vi "newmain.vi"() -> ()   [LabVIEW 2018]
uses:
  INPUTS.ctl
  <vilib>/DAQmx/read.llb/DAQmx Read (Analog 2D DBL NChan NSamp).vi
  <vilib>/DAQmx/configure/timing.llb/DAQmx Timing (Sample Clock).vi
  <vilib>/Utility/file.llb/Read Delimited Spreadsheet (DBL).vi
  <vilib>/DAQmx/miscellaneous.llb/DAQmx Fill In Error Info.vi
  <instrlib>/Kikusui PLZ 4W Series/Kikusui PLZ 4W Series.lvlib
  <instrlib>/Agilent E4360/Agilent E4360.lvlib
panel:
  out "Power":cluster{dbl[], dbl[]}[](graph) caption="VCC"
  out "P_CELL":dbl format="%0.3f"
  out "P_PV":dbl format="%0.3f"
  out "P_LOAD":dbl format="%0.3f"
  in  "DET or PPT?":enum16{"DET", "PPT"}(ring)
  out "Elapsed":dbl format="%#_13g"
  in  "SAS file":path=path "C:/Repository/bdc_prototype/logger/pcosplot.csv"
  in  "SAS VISA":refnum<visa-resource-name>="USB0::0x0957::0x1107::MY54001612::INSTR"
  in  "Load connected to?":enum16{"V_BUS", "V_CELL"}(ring)
  in  "ELO file":path=path "C:/Repository/bdc_prototype/logger/cp_profile.csv"
  in  "Serial Configuration":cluster{"Baud Rate":u32, "Stop Bits":u16}={"Baud Rate"=19200, "Stop Bits"=20} {"Stop Bits" items=["1.0"=10, "2.0"=20]; "Baud Rate" items=["2400"=2400, "4800"=4800, "9600"=9600, "19200"=19200]}
  in  "ELO VISA":refnum<visa-resource-name>="USB0::0x0B3E::0x1019::YL002399::INSTR"
  out "V_CC":dbl format="%0.3f"
  in  "Time (sec)":dbl=5560.0
  out "new file path (Not A Path if cancelled)":path
  out "I_CELL":dbl format="%0.3f"
  out "I_LOAD":dbl format="%0.3f"
  out "I_PV":dbl format="%0.3f"
  out "V_CELL":dbl format="%0.3f"
  out "V_BUS":dbl format="%0.3f"
  out "Currents":cluster{dbl[], dbl[]}[](graph) caption="VCC"
  out "Voltages":cluster{dbl[], dbl[]}[](graph) caption="VCC"
  in  "stop":bool
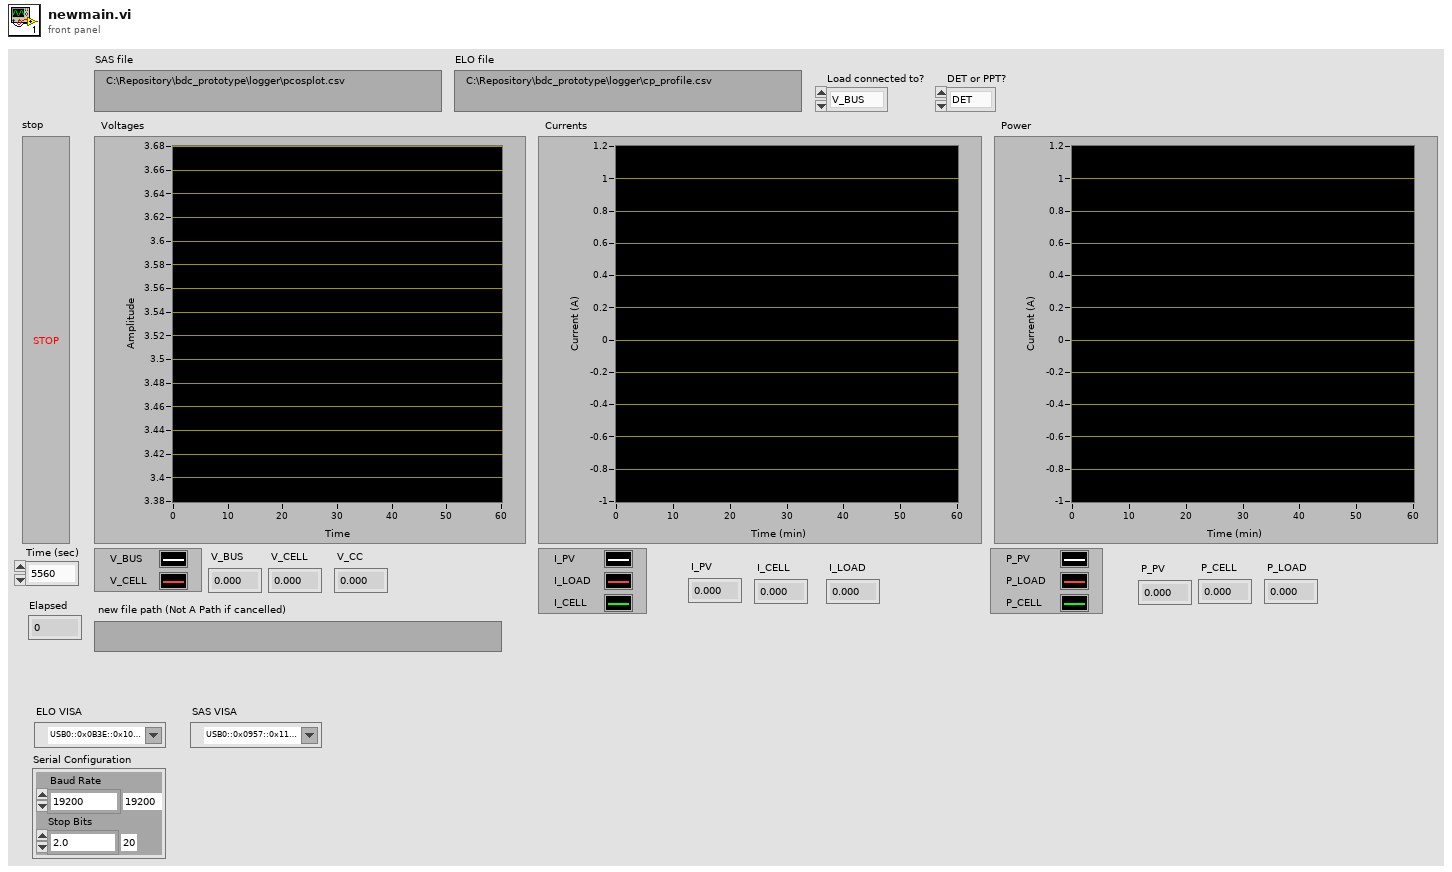
[diagram p1: front panel]
types:
  T1 = enum16{"open", "open or create", "create or replace", "create", "open (read only)"}
  T2 = typedef "INPUTS.ctl" = enum16{"VCC", "I_PV", "I_LOAD", "I_CELL", "V_BUS", "V_CELL", "I_LOAD2"}
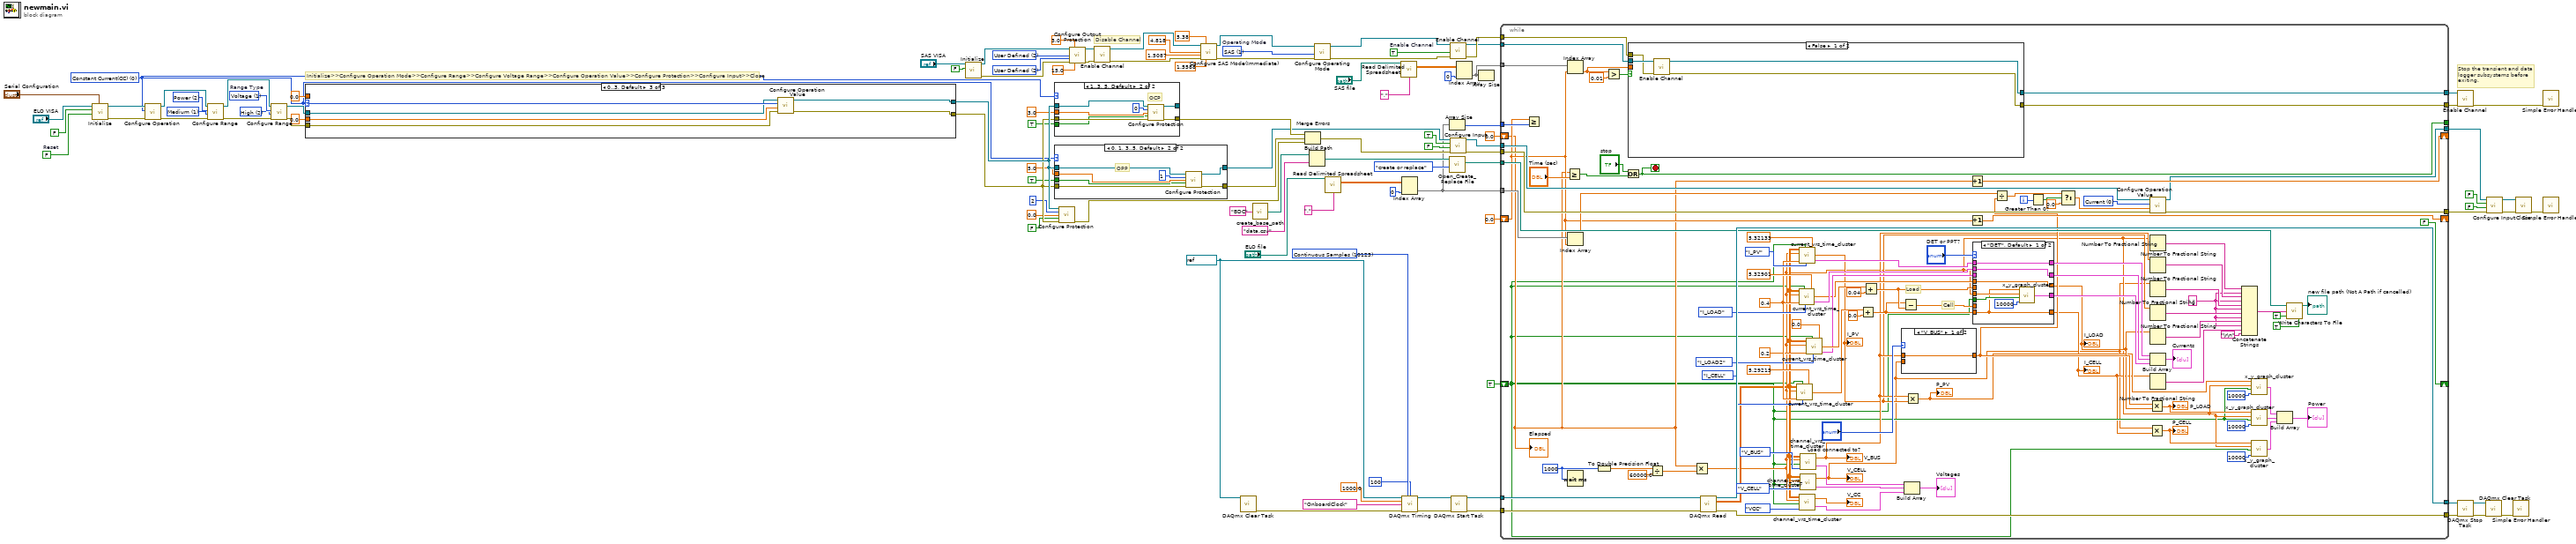
[diagram p0: block diagram]
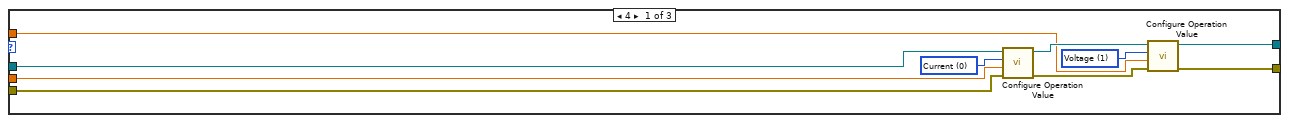
[diagram p4: hidden frame]
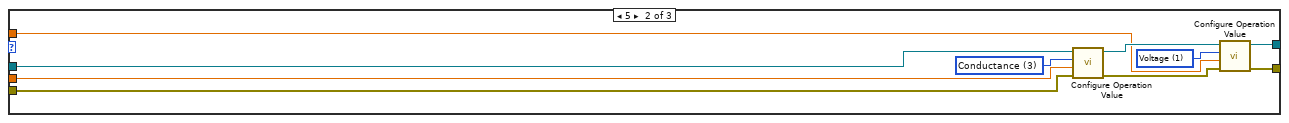
[diagram p5: hidden frame]
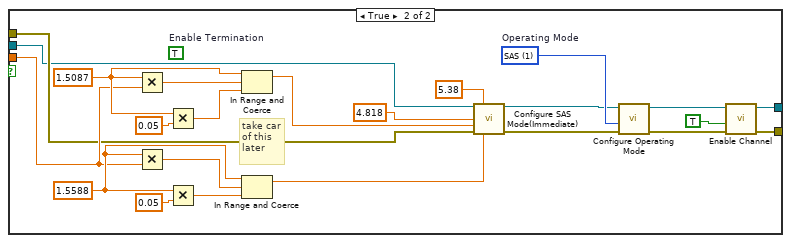
[diagram p6: hidden frame]
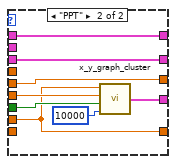
[diagram p7: hidden frame]
diagram:
  w25 = 2 items=["MAX", "MIN", "User Defined"] ("Voltage Limit Source (0:MAX)")
  w26 = 2 items=["MAX", "MIN", "User Defined"] ("Current Limit Source (0:MAX)")
  w31 = TRUE  # Enable Channel
  w32 = 1 items=["Fixed", "SAS", "Table"]  # Operating Mode
  w52 = u16 2 items=["Current", "Voltage", "Power", "Conductance"] ("Range Type (0:Current)")
  w72 = u16 2 items=["Low"=0, "High"=2] ("Voltage Range (0:Low)")
  w71 = u16 1 items=["Low", "Medium", "High"] ("Input Range (0:Low)")
  w44 = u16 0 items=["Constant Current(CC)", "Constant Voltage(CV)", "Constant Power(CP)", "Constant Resistance(CR)", "Constant Current & Voltage(CCCV)", "Constant Resistance & Voltage(CRCV)"] ("Operation Mode (0:Constant Current)")
  w56 = FALSE  # Reset
  w73 = u16 1 items=["Current", "Voltage", "Power", "Conductance"]  # Range Type
  w86 = refnum<k21> "MEAS" ("task in")
  w105 = 10123 items=["Finite Samples"=10178, "Continuous Samples"=10123, "Hardware Timed Single Point"=12522] ("sample mode")
  # "Stop the transient and data logger subsystems before exiting."
  # "Disable Channel"
  # "Initialize>>Configure Operation Mode>>Configure Range>>Configure Voltage Range>>Configure Operation Value>>Configure Protection>>Configure Input>>Close"
  n1 = call <instrlib>:"Initialize.vi"("Serial Configuration"="Serial Configuration", "Reset (True)"=w56, "ID Query (True)"=FALSE, "VISA resource name"="ELO VISA") -> ("error out"=w80:errorcluster, "VISA resource name out"=w81:refnum<visa-resource-name>)  [unwired: 6 in]
  n2 = call <instrlib>:"Configure Operation.vi"("error in (no error)"=w80, "Operation Mode (0:Constant Current)"=w44, "VISA resource name"=w81) -> ("error out"=w74:errorcluster, "VISA resource name out"=w75:refnum<visa-resource-name>)  [unwired: 7 in]
  n3 = call <instrlib>:"Configure Range.vi"("error in (no error)"=w74, "Range (0:Low)"=w71, "Range Type (0:Current)"=w52, "VISA resource name"=w75) -> ("error out"=w76:errorcluster, "VISA resource name out"=w77:refnum<visa-resource-name>)  [unwired: 6 in]
  n4 = call <instrlib>:"Configure Range.vi"("error in (no error)"=w76, "Range (0:Low)"=w72, "Range Type (0:Current)"=w73, "VISA resource name"=w77) -> ("error out"=w78:errorcluster, "VISA resource name out"=w79:refnum<visa-resource-name>)  [unwired: 6 in]
  n5 = case shown="0..3, Default" w44 {
    selector: w44 -> [_ _ w129]
    tunnel: 0.0 ("Input Value(0)") -> [w111 w119 w132]
    tunnel: w79 -> [w116 w124 w128]
    tunnel: w78 -> [w115 w123 w127]
    tunnel: [w112 w122 w131] -> w70
    tunnel: [w109 w121 w130] -> w69
    tunnel: 0.0 ("Voltage Value (0)") -> [w110 w120 _]
    frame 4 {
      w107 = u16 1 items=["Current", "Voltage", "Power", "Conductance"] ("Value Type (0:Current)")
      w108 = u16 0 items=["Current", "Voltage", "Power", "Conductance"] ("Value Type (0:Current)")
      n6 = call <instrlib>:"Configure Operation Value.vi"("error in (no error)"=w115, "Values (0)"=w111, "Value Type (0:Current)"=w108, "VISA resource name"=w116) -> ("error out"=w113:errorcluster, "VISA resource name out"=w114:refnum<visa-resource-name>)  [unwired: 6 in]
      n7 = call <instrlib>:"Configure Operation Value.vi"("error in (no error)"=w113, "Values (0)"=w110, "Value Type (0:Current)"=w107, "VISA resource name"=w114) -> ("error out"=w109:errorcluster, "VISA resource name out"=w112:refnum<visa-resource-name>)  [unwired: 6 in]
    }
    frame 5 {
      w117 = u16 1 items=["Current", "Voltage", "Power", "Conductance"] ("Value Type (0:Current)")
      w118 = u16 3 items=["Current", "Voltage", "Power", "Conductance"] ("Value Type (0:Current)")
      n8 = call <instrlib>:"Configure Operation Value.vi"("error in (no error)"=w123, "Values (0)"=w119, "Value Type (0:Current)"=w118, "VISA resource name"=w124) -> ("error out"=w125:errorcluster, "VISA resource name out"=w126:refnum<visa-resource-name>)  [unwired: 6 in]
      n9 = call <instrlib>:"Configure Operation Value.vi"("error in (no error)"=w125, "Values (0)"=w120, "Value Type (0:Current)"=w117, "VISA resource name"=w126) -> ("error out"=w121:errorcluster, "VISA resource name out"=w122:refnum<visa-resource-name>)  [unwired: 6 in]
    }
    frame 0..3, Default {
      n10 = call <instrlib>:"Configure Operation Value.vi"("error in (no error)"=w127, "Values (0)"=w132, "Value Type (0:Current)"=w129, "VISA resource name"=w128) -> ("error out"=w130:errorcluster, "VISA resource name out"=w131:refnum<visa-resource-name>)  [unwired: 6 in]
    }
  }
  n11 = call <instrlib>:"Initialize.vi"("ID Query (True)"=FALSE, "VISA resource name"="SAS VISA") -> ("error out"=w29:errorcluster, "VISA resource name out"=w30:refnum<visa-resource-name>)  [unwired: 8 in]
  n12 = case shown="1..3, 5, Default" w44 {
    tunnel: w70 -> [w134 w141]
    tunnel: w69 -> [w133 w140]
    tunnel: [w134 w139] -> _
    tunnel: [w133 w138] -> w68
    tunnel: 3.0 ("OCP Limit (0)") -> [_ w137]
    tunnel: TRUE ("OCP Trip (Disable)") -> [_ w135]
    frame 0, 4 {
    }
    frame 1..3, 5, Default {
      # "OCP"
      n13 = call <instrlib>:"Configure Protection.vi"("VISA resource name"=w141, "Protection Type (0:OCP)"=0, "Protection Limit (0)"=w137, "Enable Trip (Disable)"=w135, "error in (no error)"=w140) -> ("VISA resource name out"=w139:refnum<visa-resource-name>, "error out"=w138:errorcluster)  [unwired: 9 in]
    }
  }
  n14 = case shown="0, 1, 3..5, Default" w44 {
    tunnel: w70 -> [w143 w150]
    tunnel: w69 -> [w142 w149]
    tunnel: [w143 w148] -> w65
    tunnel: [w142 w147] -> w58
    tunnel: 5.0 ("OPP Limit (0)") -> [_ w146]
    tunnel: TRUE ("OPP Trip (Disable)") -> [_ w144]
    frame 2 {
    }
    frame 0, 1, 3..5, Default {
      # "OPP"
      n15 = call <instrlib>:"Configure Protection.vi"("VISA resource name"=w150, "Protection Type (0:OCP)"=1, "Protection Limit (0)"=w146, "Enable Trip (Disable)"=w144, "error in (no error)"=w149) -> ("VISA resource name out"=w148:refnum<visa-resource-name>, "error out"=w147:errorcluster)  [unwired: 9 in]
    }
  }
  n16 = call <instrlib>:"Configure Protection.vi"("VISA resource name"=w70, "Protection Type (0:OCP)"=2, "Protection Limit (0)"=0.0 ("UVP Limit (0)"), "Enable Trip (Disable)"=FALSE ("UVP (Enable)"), "error in (no error)"=w69) -> ("error out"=w67:errorcluster)  [unwired: 9 in, 1 out]
  n17 = call <instrlib>:"Configure Output Protection.vi"("VISA resource name"=w30, "Current Limit (0 A)"=3.0, "Current Limit Source (0:MAX)"=w26, "Voltage Limit Source (0:MAX)"=w25, "error in (no error)"=w29, "Voltage Limit (0 V)"=15.0) -> ("VISA resource name out"=w16:refnum<visa-resource-name>, "error out"=w15:errorcluster)  [unwired: 8 in]
  n18 = call <instrlib>:"Enable Channel.vi"("error in (no error)"=w15, "VISA resource name"=w16) -> ("error out"=w23:errorcluster, "VISA resource name out"=w24:refnum<visa-resource-name>)  [unwired: 8 in]
  n19 = call <instrlib>:"Configure SAS Mode(Immediate).vi"("VISA resource name"=w24, "Open Circuit Voltage (0.0 V)"=5.38, "Maximum Voltage Point (0.0 V)"=4.818, "Maximum Current Point (0.0 A)"=1.5087, "error in (no error)"=w23, "Short Circuit Current (0.0 A)"=1.5588) -> ("VISA resource name out"=w18:refnum<visa-resource-name>, "error out"=w17:errorcluster)  [unwired: 8 in]
  n20 = call <vilib>:"DAQmx Clear Task.vi"("task in"=w86) -> ("error out"=w85:errorcluster)  [unwired: 14 in]
  n21 = call "create_base_path.vi"("project name"="BDC") -> ("base path"=w89:path)
  n22 = Merge Errors(w68, w58, w67) -> (w66:errorcluster)
  n23 = Build Path(base path=w89, name or relative path="data.csv") -> (appended path=w91:path)
  n24 = call <instrlib>:"Configure Operating Mode.vi"("error in (no error)"=w17, "Operating Mode (0:Fixed)"=w32, "VISA resource name"=w18) -> ("error out"=w13:errorcluster, "VISA resource name out"=w14:refnum<visa-resource-name>)  [unwired: 7 in]
  n25 = call-poly <vilib>:"Read Delimited Spreadsheet.vi"("file path (dialog if empty)"="ELO file", "delimiter (\\t)"="," ("delimiter (\\t)")) -> ("all rows"=w47:dbl[][])  [unwired: 8 in, 5 out]
  n26 = call-poly <vilib>:"Read Delimited Spreadsheet.vi"("file path (dialog if empty)"="SAS file", "delimiter (\\t)"="," ("delimiter (\\t)")) -> ("all rows"=w8:dbl[][])  [unwired: 8 in, 5 out]
  n27 = Index Array(array=w47, index (col)=0 ("disabled index (col)")) -> (element=w43:dbl[])  [unwired: 1 in]
  n28 = call-poly <vilib>:"DAQmx Timing.vi"("task/channels in"=w86, "sample mode"=w105, "samples per channel"=100, "rate"=1000.0, "source"=tag "OnboardClock", "error in"=w85) -> ("task out"=w102:refnum<k21>, "error out"=w101:errorcluster)  [unwired: 8 in]
  n29 = Array Size(array=w43) -> (size(s)=w42:i32)
  n30 = call <vilib>:"Open_Create_Replace File.vi"("function (open:0)"=T1."create or replace", "file path"=w91) -> ("new file path"=w87:path)  [unwired: 6 in, 3 out]
  n31 = call <instrlib>:"Enable Channel.vi"("error in (no error)"=w13, "Enable Channel (Disable)"=w31, "VISA resource name"=w14) -> ("error out"=w6:errorcluster, "VISA resource name out"=w5:refnum<visa-resource-name>)  [unwired: 7 in]
  n32 = call <instrlib>:"Configure Input.vi"("error in (no error)"=w66, "Enable Input Short (Disable)"=FALSE, "Enable Input (Enable)"=TRUE, "VISA resource name"=w65) -> ("error out"=w45:errorcluster, "VISA resource name out"=w46:refnum<visa-resource-name>)  [unwired: 6 in]
  n33 = call <vilib>:"DAQmx Start Task.vi"("task/channels in"=w102, "error in"=w101) -> ("task out"=w100:refnum<k21>, "error out"=w99:errorcluster)  [unwired: 12 in]
  n34 = Index Array(array=w8, index (col)=0 ("disabled index (col)")) -> (element=w7:dbl[])  [unwired: 1 in]
  n35 = Array Size(array=w7) -> ()  [unwired: 1 out]
  n36 = while {
    shift-right: [w224] -> _
    shift-left: 0.0 -> [w172]
    shift-right: [FALSE ("Clear Graph?")] -> _
    shift-left: TRUE ("Clear Graph?") -> [w155]
    tunnel: w100 -> [w250]
    tunnel: w99 -> [w249]
    tunnel: [w248] -> w98
    tunnel: [w247] -> w97
    tunnel: w87 -> [w225]
    tunnel: [w218] -> _
    tunnel: w46 -> [w209]
    tunnel: w45 -> [w208]
    tunnel: w43 -> [w207]
    tunnel: w42 -> [w206]
    tunnel: [w205] -> w36
    tunnel: [w204] -> w35
    shift-right: [w196] -> _
    shift-left: 0.0 -> [w194]
    tunnel: w7 -> [w195]
    tunnel: w6 -> [w193]
    tunnel: w5 -> [w192]
    tunnel: [w191] -> w3
    tunnel: [w190] -> w2
    i -> [w198]
    stop <- w218 stop-if-true
    w210 = u16 0 items=["Current", "Voltage", "Power", "Conductance"] ("Value Type (0:Current)")
    w228 = "," ("string")
    w211 = 0.4 ("sensitivity (V/A)")
    w251 = u32 1000 ("milliseconds to wait")
    # "Cell"
    # "Load"
    n37 = Greater Or Equal?(x=w194, y=w206) -> ()  [unwired: 1 out]
    n38 = Greater Or Equal?(x=w172, y="Time (sec)") -> (x >= y?=w219:bool)
    n39 = Index Array(array=w195, index=w194) -> (element=w170:dbl)
    n40 = Index Array(array=w207, index=w194) -> (element=w203:dbl)
    n41 = Wait (ms)(milliseconds to wait=w251) -> ()  [unwired: 1 out]
    n42 = To Double Precision Float(number=w251) -> (double precision float=w254:dbl)
    n43 = Greater?(x=w170, y=0.01) -> (0:w169:bool)
    n44 = Or(x="stop", y=w219) -> (x .or. y?=w218:bool)
    n45 = case shown="False" w169 {
      tunnel: w170 -> [_ w264]
      tunnel: w193 -> [w258 w263]
      tunnel: w192 -> [w259 w262]
      tunnel: [w257 w261] -> w191
      tunnel: [w256 w260] -> w190
      frame False {
        n46 = call <instrlib>:"Enable Channel.vi"("error in (no error)"=w258, "VISA resource name"=w259) -> ("error out"=w256:errorcluster, "VISA resource name out"=w257:refnum<visa-resource-name>)  [unwired: 8 in]
      }
      frame True {
        w274 = 1 items=["Fixed", "SAS", "Table"]  # Operating Mode
        w265 = 1.5588 ("Maximum Current Point (0.0 A)")
        w266 = 1.5087 ("Maximum Current Point (0.0 A)")
        (unwired) TRUE  # Enable Termination
        # "take car\nof this \nlater"
        n47 = Multiply(x=w266, y=w264) -> (x*y=w268:dbl)
        n48 = Multiply(x=w265, y=w264) -> (x*y=w267:dbl)
        n49 = Multiply(x=w266, y=0.05) -> (x*y=w278:dbl)
        n50 = Multiply(x=w265, y=0.05) -> (x*y=w276:dbl)
        n51 = In Range and Coerce(upper limit=w266, x=w268, lower limit=w278) -> (coerced(x)=w280:dbl)  [unwired: 1 out]
        n52 = In Range and Coerce(upper limit=w265, x=w267, lower limit=w276) -> (coerced(x)=w275:dbl)  [unwired: 1 out]
        n53 = call <instrlib>:"Configure SAS Mode(Immediate).vi"("VISA resource name"=w262, "Open Circuit Voltage (0.0 V)"=5.38, "Maximum Voltage Point (0.0 V)"=4.818, "Maximum Current Point (0.0 A)"=w280, "error in (no error)"=w263, "Short Circuit Current (0.0 A)"=w275) -> ("VISA resource name out"=w273:refnum<visa-resource-name>, "error out"=w272:errorcluster)  [unwired: 8 in]
        n54 = call <instrlib>:"Configure Operating Mode.vi"("error in (no error)"=w272, "Operating Mode (0:Fixed)"=w274, "VISA resource name"=w273) -> ("error out"=w270:errorcluster, "VISA resource name out"=w271:refnum<visa-resource-name>)  [unwired: 7 in]
        n55 = call <instrlib>:"Enable Channel.vi"("error in (no error)"=w270, "Enable Channel (Disable)"=TRUE, "VISA resource name"=w271) -> ("error out"=w260:errorcluster, "VISA resource name out"=w261:refnum<visa-resource-name>)  [unwired: 7 in]
      }
    }
    n56 = Divide(x=w254, y=60000.0) -> (x/y=w252:dbl)
    n57 = Multiply(x=w172, y=w252) -> (x*y=w156:dbl)
    n58 = call-poly <vilib>:"DAQmx Read.vi"("task/channels in"=w250, "error in"=w249) -> ("task out"=w248:refnum<k21>, "data"=w184:dbl[][], "error out"=w247:errorcluster)  [unwired: 11 in]
    n59 = call "current_vrs_time_cluster.vi"("Input data"=w184, "Clear Graph?"=w155, "Time"=w156, 4:INPUTS."I_CELL", "sensitivity (V/A)"=w211, "VCC"=5.29215) -> ("rms value"=w213:dbl)  [unwired: 1 in, 1 out]
    n60 = call "current_vrs_time_cluster.vi"("Input data"=w184, "Clear Graph?"=w155, "Time"=w156, 4:INPUTS."I_LOAD", "sensitivity (V/A)"=w211, "VCC"=5.32901) -> ("rms value"=w176:dbl, "Cluster"=w180:cluster{dbl[], dbl[]})  [unwired: 1 in]
    n61 = call "current_vrs_time_cluster.vi"("Input data"=w184, "Clear Graph?"=w155, "Time"=w156, 4:INPUTS."I_PV", "sensitivity (V/A)"=w211, "VCC"=5.32133) -> ("rms value"=w162:dbl, "Cluster"=w183:cluster{dbl[], dbl[]})  [unwired: 1 in]
    "I_PV" <- w162
    n62 = call "channel_vrs_time_cluster.vi"(2:INPUTS."VCC", "Clear Graph?"=w155, "Time"=w156, "Input data"=w184) -> ("Cluster"=w242:cluster{dbl[], dbl[]}, "rms value"=→"V_CC":dbl)
    n63 = call "channel_vrs_time_cluster.vi"(2:INPUTS."V_BUS", "Clear Graph?"=w155, "Time"=w156, "Input data"=w184) -> ("Cluster"=w245:cluster{dbl[], dbl[]}, "rms value"=w163:dbl)
    "V_BUS" <- w163
    n64 = call "channel_vrs_time_cluster.vi"(2:INPUTS."V_CELL", "Clear Graph?"=w155, "Time"=w156, "Input data"=w184) -> ("Cluster"=w244:cluster{dbl[], dbl[]}, "rms value"=w153:dbl)
    "V_CELL" <- w153
    n65 = call "current_vrs_time_cluster.vi"("Input data"=w184, "Clear Graph?"=w155, "Time"=w156, 4:INPUTS."I_LOAD2", "sensitivity (V/A)"=0.2, "VCC"=0.0) -> ("rms value"=w186:dbl, "Cluster"=w177:cluster{dbl[], dbl[]})  [unwired: 1 in]
    n66 = Add(x=w213, y=0.0) -> (x+y=w174:dbl)
    n67 = Add(x=w186, y=0.04) -> (x+y=w175:dbl)
    n68 = case shown="\"V_BUS\"" "Load connected to?" {
      tunnel: w163 -> [w299 _]
      tunnel: [w299 w300] -> w168
      tunnel: w153 -> [_ w300]
      frame "V_BUS" {
      }
      frame "V_CELL" {
      }
    }
    n69 = Subtract(x=w174, y=w175) -> (x-y=w173:dbl)
    n70 = Build Array(w245, w244, w242) -> (→"Voltages":cluster{dbl[], dbl[]}[])
    n71 = Multiply(x=w163, y=w162) -> (x*y=w158:dbl)
    "P_PV" <- w158
    n72 = Increment(x=w172) -> (x+1=w224:dbl)
    n73 = Increment(x=w194) -> (x+1=w196:dbl)
    n74 = case shown="\"DET\", Default" "DET or PPT?" {
      tunnel: w183 -> [w290 w298]
      tunnel: [w290 w298] -> w182
      tunnel: w180 -> [w289 _]
      tunnel: [w289 w297] -> w179
      tunnel: [w283 w291] -> w178
      tunnel: w177 -> [_ w297]
      tunnel: w176 -> [w288 _]
      tunnel: [w288 w296] -> w167
      tunnel: w175 -> [_ w296]
      tunnel: w174 -> [w284 _]
      tunnel: [w284 w292] -> w154
      tunnel: w173 -> [_ w292]
      tunnel: w155 -> [w286 w294]
      tunnel: w156 -> [w285 w293]
      frame "DET", Default {
        n75 = call "x_y_graph_cluster.vi"("Chart History (10,000)"=10000, "Clear Graph?"=w286, "X"=w285, "Y"=w284) -> ("Cluster"=w283:cluster{dbl[], dbl[]})
      }
      frame "PPT" {
        n76 = call "x_y_graph_cluster.vi"("Chart History (10,000)"=10000, "Clear Graph?"=w294, "X"=w293, "Y"=w292) -> ("Cluster"=w291:cluster{dbl[], dbl[]})
      }
    }
    "I_LOAD" <- w167
    "I_CELL" <- w154
    n77 = Divide(x=w203, y=w168) -> (x/y=w201:dbl)
    n78 = Greater Than 0?(x=w198) -> (x > 0?=w197:bool)
    n79 = Select(t=w201, s=w197, f=0.0) -> (s? t:f=w200:dbl)
    n80 = Multiply(x=w168, y=w167) -> (x*y=w160:dbl)
    "P_LOAD" <- w160
    n81 = Multiply(x=w153, y=w154) -> (x*y=w157:dbl)
    "P_CELL" <- w157
    n82 = call <instrlib>:"Configure Operation Value.vi"("error in (no error)"=w208, "Values (0)"=w200, "Value Type (0:Current)"=w210, "VISA resource name"=w209) -> ("error out"=w204:errorcluster, "VISA resource name out"=w205:refnum<visa-resource-name>)  [unwired: 6 in]
    n83 = Number To Fractional String(number=w156) -> (F-format string=w234:string)  [unwired: 3 in]
    n84 = Number To Fractional String(number=w163) -> (F-format string=w232:string)  [unwired: 3 in]
    n85 = Number To Fractional String(number=w153) -> (F-format string=w231:string)  [unwired: 3 in]
    n86 = Number To Fractional String(number=w162) -> (F-format string=w230:string)  [unwired: 3 in]
    n87 = Number To Fractional String(number=w167) -> (F-format string=w229:string)  [unwired: 3 in]
    n88 = Build Array(w182, w179, w178) -> (→"Currents":cluster{dbl[], dbl[]}[])
    n89 = Number To Fractional String(number=w154) -> (F-format string=w227:string)  [unwired: 3 in]
    n90 = Concatenate Strings(w234, w228, w232, w228, w231, w228, w230, w228, w229, w228, w227, "\r\n") -> (w233:string)
    n91 = call "x_y_graph_cluster.vi"("Chart History (10,000)"=10000, "Clear Graph?"=w155, "X"=w156, "Y"=w158) -> ("Cluster"=w161:cluster{dbl[], dbl[]})
    n92 = call "x_y_graph_cluster.vi"("Chart History (10,000)"=10000, "Clear Graph?"=w155, "X"=w156, "Y"=w160) -> ("Cluster"=w165:cluster{dbl[], dbl[]})
    n93 = call "x_y_graph_cluster.vi"("Chart History (10,000)"=10000, "Clear Graph?"=w155, "X"=w156, "Y"=w157) -> ("Cluster"=w152:cluster{dbl[], dbl[]})
    n94 = Build Array(w161, w165, w152) -> (→"Power":cluster{dbl[], dbl[]}[])
    n95 = call <vilib>:"Write Characters To File.vi"("convert eol? (no:F)"=TRUE, "append to file? (new file:F)"=TRUE, "character string"=w233, "file path (dialog if empty)"=w225) -> ("new file path (Not A Path if cancelled)"=→"new file path (Not A Path if cancelled)":path)  [unwired: 1 in]
    "Elapsed" <- w172
  }
  n96 = call <instrlib>:"Enable Channel.vi"("error in (no error)"=w2, "VISA resource name"=w3) -> ("error out"=w4:errorcluster)  [unwired: 8 in, 1 out]
  n97 = call <vilib>:"DAQmx Stop Task.vi"("task/channels in"=w98, "error in"=w97) -> ("task out"=w96:refnum<k21>, "error out"=w95:errorcluster)  [unwired: 12 in]
  n98 = call <vilib>:"DAQmx Clear Task.vi"("task in"=w96, "error in"=w95) -> ("error out"=w94:errorcluster)  [unwired: 13 in]
  n99 = call <instrlib>:"Configure Input.vi"("error in (no error)"=w35, "Enable Input Short (Disable)"=FALSE ("Enable Input Short (Disable) 2"), "Enable Input (Enable)"=FALSE ("Enable Input (Enable) 2"), "VISA resource name"=w36) -> ("error out"=w37:errorcluster, "VISA resource name out"=w38:refnum<visa-resource-name>)  [unwired: 6 in]
  n100 = call <vilib>:"Simple Error Handler.vi"("error in (no error)"=w94) -> ()  [unwired: 4 in, 5 out]
  n101 = call <instrlib>:"Close.vi"("error in (no error)"=w37, "VISA resource name"=w38) -> ("error out"=w41:errorcluster)  [unwired: 9 in]
  n102 = call <vilib>:"Simple Error Handler.vi"("error in (no error)"=w4) -> ()  [unwired: 4 in, 5 out]
  n103 = call <vilib>:"Simple Error Handler.vi"("error in (no error)"=w41) -> ()  [unwired: 4 in, 5 out]
